vi "SW_Load_settings_to_main_tab_2.vi"(0 "Settings path in":path, 2 "Researcher name":string="Researcher", 3 "error in (no error)":errorcluster) -> (6 "Settings cluster out":T1={"Defaults"={"Default User"=0.0, "VISA Resource Name "=""}, "Recording and saving"={"Researcher name"="", "Name prefix"="", "Data filtering"=0, "Stop at"=0.0, "\"Stop at\" enabled"=FALSE}, "Geometry"={"Cage diameter, mm"=0, "Starting angle MIDFIELD"=0, "Starting angle BORDER"=0, "Radius, mm CENTER"=0, "Radius, mm MIDFIELD"=0, "N segments MIDFIELD"=0, "N segments BORDER"=0, "R-gap, mm"=0.0, "Bridge swap"=FALSE, "Bridge H. offset"=0.0, "Bridge V. offset"=0.0, "Twisted neck"=FALSE}, "IO parameters"={"IO general config."=0, "IO 1 configuration"=0, "IO 2 configuration"=0, "IO 3 configuration"=0, "IO 4 configuration"=0, "Activate ext. RS-232"=0, "IO inversion config."=0, "Sync capability"=1}, "Stimulus presets array"=[{"Event type"=0, "Dur., s"=0.0, "Stim., s"=0.0, "TTL out N"=1, "Set/Clear"=FALSE, "Stim. has been set"=FALSE}, {"Event type"=0, "Dur., s"=0.0, "Stim., s"=0.0, "TTL out N"=1, "Set/Clear"=FALSE, "Stim. has been set"=FALSE}, {"Event type"=0, "Dur., s"=0.0, "Stim., s"=0.0, "TTL out N"=1, "Set/Clear"=FALSE, "Stim. has been set"=FALSE}, {"Event type"=0, "Dur., s"=0.0, "Stim., s"=0.0, "TTL out N"=1, "Set/Clear"=FALSE, "Stim. has been set"=FALSE}, {"Event type"=0, "Dur., s"=0.0, "Stim., s"=0.0, "TTL out N"=1, "Set/Clear"=FALSE, "Stim. has been set"=FALSE}, {"Event type"=0, "Dur., s"=0.0, "Stim., s"=0.0, "TTL out N"=1, "Set/Clear"=FALSE, "Stim. has been set"=FALSE}, {"Event type"=0, "Dur., s"=0.0, "Stim., s"=0.0, "TTL out N"=1, "Set/Clear"=FALSE, "Stim. has been set"=FALSE}, {"Event type"=0, "Dur., s"=0.0, "Stim., s"=0.0, "TTL out N"=1, "Set/Clear"=FALSE, "Stim. has been set"=FALSE}, {"Event type"=0, "Dur., s"=0.0, "Stim., s"=0.0, "TTL out N"=1, "Set/Clear"=FALSE, "Stim. has been set"=FALSE}, {"Event type"=0, "Dur., s"=0.0, "Stim., s"=0.0, "TTL out N"=1, "Set/Clear"=FALSE, "Stim. has been set"=FALSE}, {"Event type"=0, "Dur., s"=0.0, "Stim., s"=0.0, "TTL out N"=1, "Set/Clear"=FALSE, "Stim. has been set"=FALSE}, {"Event type"=0, "Dur., s"=0.0, "Stim., s"=0.0, "TTL out N"=1, "Set/Clear"=FALSE, "Stim. has been set"=FALSE}, {"Event type"=0, "Dur., s"=0.0, "Stim., s"=0.0, "TTL out N"=1, "Set/Clear"=FALSE, "Stim. has been set"=FALSE}, {"Event type"=0, "Dur., s"=0.0, "Stim., s"=0.0, "TTL out N"=1, "Set/Clear"=FALSE, "Stim. has been set"=FALSE}], "Settings loaded OK"=FALSE} {"Stimulus presets array"."Event type" items=["Stay for N seconds"]; "Stimulus presets array"."TTL out N" items=["1"=1, "2"=2, "1+2"=3]; "Geometry"."Cage diameter, mm" scale=0.0..340.0}, 7 "Settings file path":path, 10 "error out":errorcluster={"status"=TRUE, "code"=1, "source"="Dequeue Element in NI_LVConfig.lvlib:Read Value Without Comment.vi->NI_LVConfig.lvlib:Read Key (I32).vi->SW_Load_settings_to_main_tab.vi"})   [LabVIEW 2018]
uses:
  Controls/CTL_Settings_cluster.ctl
  Controls/CTL_IO_params_cluster.ctl
  Controls/CTL_Single_stimulus_setting.ctl
  <vilib>/Utility/config.llb/NI_LVConfig.lvlib
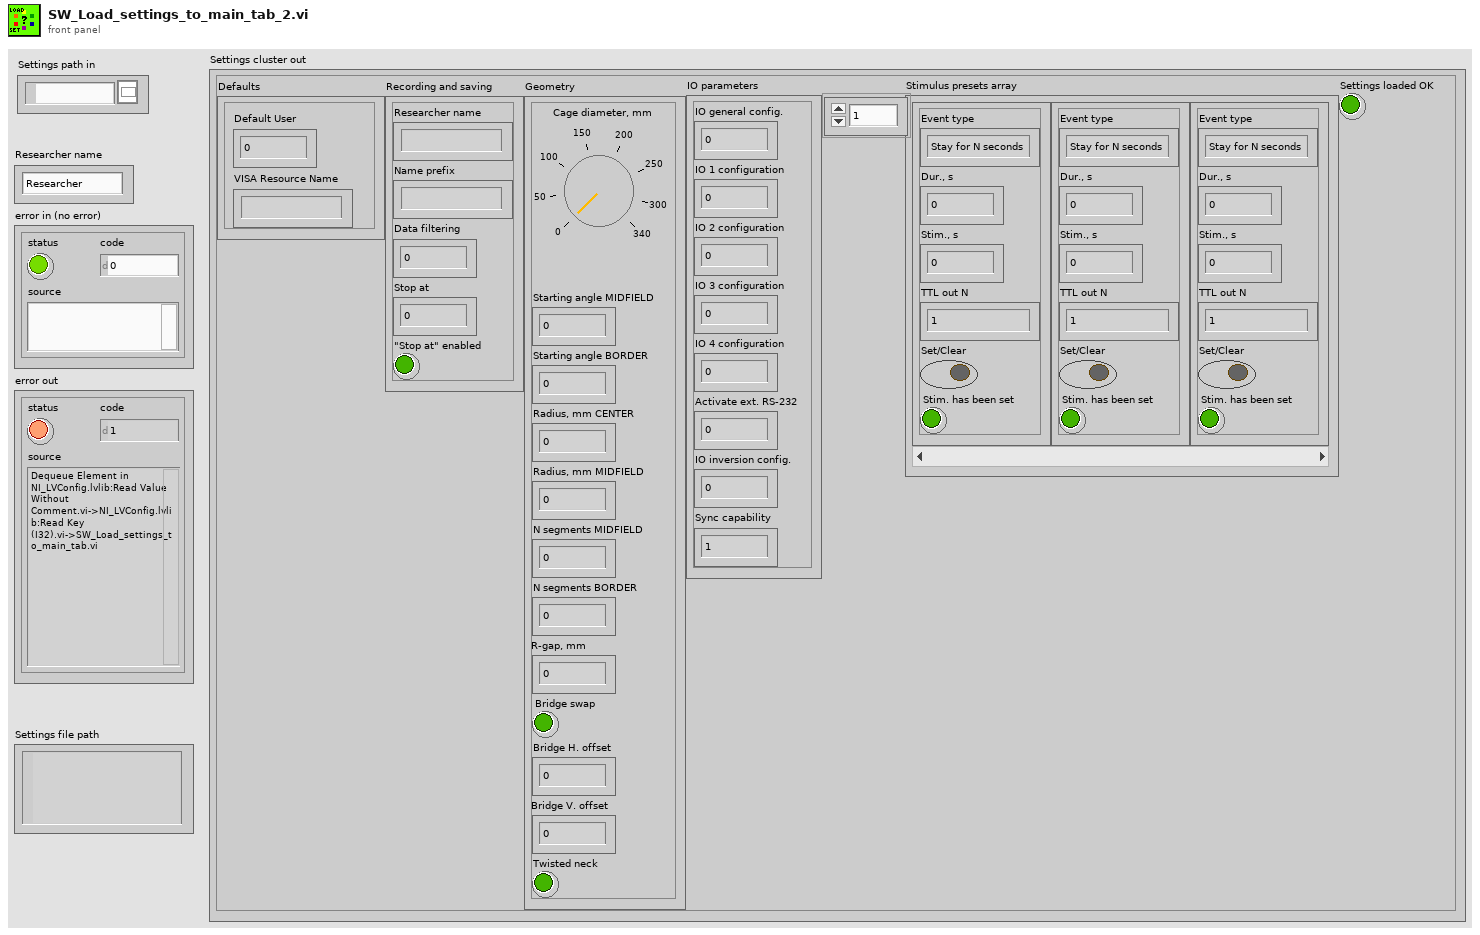
[diagram p1: front panel]
types:
  T1 = typedef "CTL_Settings_cluster.ctl" = cluster{"Defaults":cluster{"Default User":dbl, "VISA Resource Name ":string}, "Recording and saving":cluster{"Researcher name":string, "Name prefix":string, "Data filtering":u16, "Stop at":dbl, "\"Stop at\" enabled":bool}, "Geometry":cluster{"Cage diameter, mm":u16, "Starting angle MIDFIELD":i16, "Starting angle BORDER":i16, "Radius, mm CENTER":u16, "Radius, mm MIDFIELD":u16, "N segments MIDFIELD":u8, "N segments BORDER":u8, "R-gap, mm":sgl, "Bridge swap":bool, "Bridge H. offset":sgl, "Bridge V. offset":sgl, "Twisted neck":bool}, "IO parameters":T2, "Stimulus presets array":T3[], "Settings loaded OK":bool}
  T2 = typedef "CTL_IO_params_cluster.ctl" = cluster{"IO general config.":u16, "IO 1 configuration":u16, "IO 2 configuration":u16, "IO 3 configuration":u16, "IO 4 configuration":u16, "Activate ext. RS-232":u16, "IO inversion config.":u16, "Sync capability":u8}
  T3 = typedef "CTL_Single_stimulus_setting.ctl" = cluster{"Event type":u16, "Dur., s":sgl, "Stim., s":sgl, "TTL out N":u16, "Set/Clear":bool, "Stim. has been set":bool}
  T4 = typedef "NI_LVConfig.lvlib/Config Data RefNum.ctl" = refnum<k1>
  T5 = cluster{"Default User":dbl, "VISA Resource Name ":string}
  T6 = cluster{"Researcher name":string, "Name prefix":string, "Data filtering":u16, "Stop at":dbl, "\"Stop at\" enabled":bool}
  T7 = cluster{"Cage diameter, mm":u16, "Starting angle MIDFIELD":i16, "Starting angle BORDER":i16, "Radius, mm CENTER":u16, "Radius, mm MIDFIELD":u16, "N segments MIDFIELD":u8, "N segments BORDER":u8, "R-gap, mm":sgl, "Bridge swap":bool, "Bridge H. offset":sgl, "Bridge V. offset":sgl, "Twisted neck":bool}
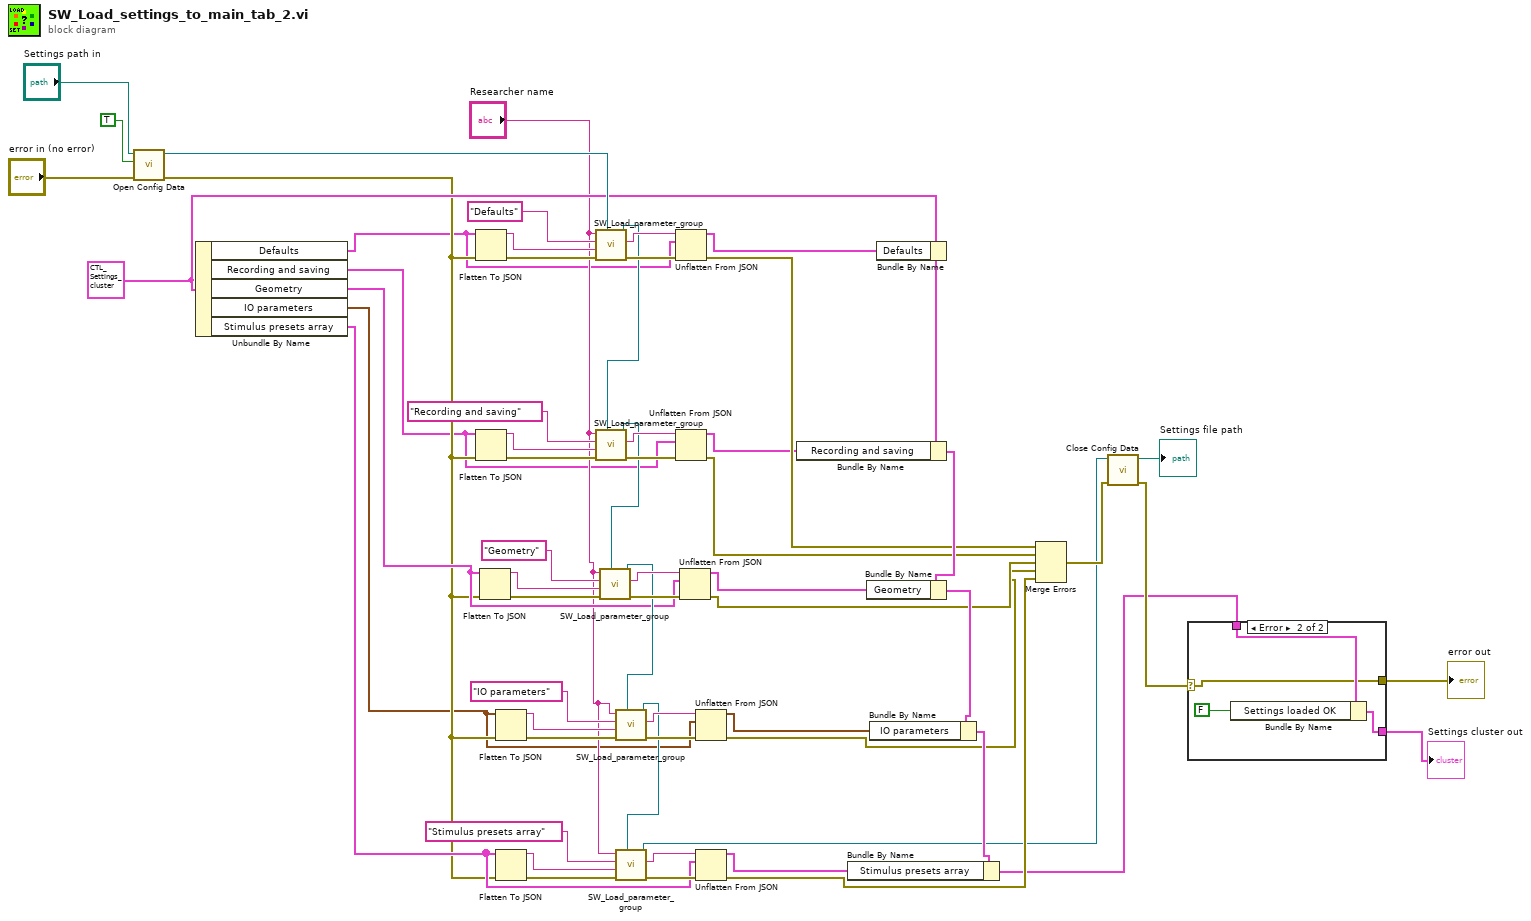
[diagram p0: block diagram]
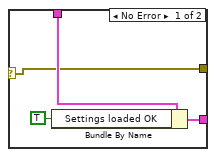
[diagram p2: hidden frame]
diagram:
  w39 = T1 {"Defaults"={"Default User"=0.0, "VISA Resource Name "="Tracker"}, "Recording and saving"={"Researcher name"="Researcher", "Name prefix"="Track", "Data filtering"=5, "Stop at"=0.0, "\"Stop at\" enabled"=FALSE}, "Geometry"={"Cage diameter, mm"=180, "Starting angle MIDFIELD"=0, "Starting angle BORDER"=0, "Radius, mm CENTER"=30, "Radius, mm MIDFIELD"=75, "N segments MIDFIELD"=2, "N segments BORDER"=4, "R-gap, mm"=0.0, "Bridge swap"=FALSE, "Bridge H. offset"=0.0, "Bridge V. offset"=0.0, "Twisted neck"=FALSE}, "IO parameters"={"IO general config."=12, "IO 1 configuration"=1, "IO 2 configuration"=1, "IO 3 configuration"=0, "IO 4 configuration"=0, "Activate ext. RS-232"=0, "IO inversion config."=0, "Sync capability"=1}, "Stimulus presets array"=[{"Event type"=0, "Dur., s"=0.0, "Stim., s"=0.0, "TTL out N"=1, "Set/Clear"=FALSE, "Stim. has been set"=FALSE}, {"Event type"=0, "Dur., s"=0.0, "Stim., s"=0.0, "TTL out N"=1, "Set/Clear"=FALSE, "Stim. has been set"=FALSE}, {"Event type"=0, "Dur., s"=0.0, "Stim., s"=0.0, "TTL out N"=1, "Set/Clear"=FALSE, "Stim. has been set"=FALSE}, {"Event type"=0, "Dur., s"=0.0, "Stim., s"=0.0, "TTL out N"=1, "Set/Clear"=FALSE, "Stim. has been set"=FALSE}, {"Event type"=0, "Dur., s"=0.0, "Stim., s"=0.0, "TTL out N"=1, "Set/Clear"=FALSE, "Stim. has been set"=FALSE}, {"Event type"=0, "Dur., s"=0.0, "Stim., s"=0.0, "TTL out N"=1, "Set/Clear"=FALSE, "Stim. has been set"=FALSE}, {"Event type"=0, "Dur., s"=0.0, "Stim., s"=0.0, "TTL out N"=1, "Set/Clear"=FALSE, "Stim. has been set"=FALSE}, {"Event type"=0, "Dur., s"=0.0, "Stim., s"=0.0, "TTL out N"=1, "Set/Clear"=FALSE, "Stim. has been set"=FALSE}, {"Event type"=0, "Dur., s"=0.0, "Stim., s"=0.0, "TTL out N"=1, "Set/Clear"=FALSE, "Stim. has been set"=FALSE}, {"Event type"=0, "Dur., s"=0.0, "Stim., s"=0.0, "TTL out N"=1, "Set/Clear"=FALSE, "Stim. has been set"=FALSE}, {"Event type"=0, "Dur., s"=0.0, "Stim., s"=0.0, "TTL out N"=1, "Set/Clear"=FALSE, "Stim. has been set"=FALSE}, {"Event type"=0, "Dur., s"=0.0, "Stim., s"=0.0, "TTL out N"=1, "Set/Clear"=FALSE, "Stim. has been set"=FALSE}, {"Event type"=0, "Dur., s"=0.0, "Stim., s"=0.0, "TTL out N"=1, "Set/Clear"=FALSE, "Stim. has been set"=FALSE}, {"Event type"=0, "Dur., s"=0.0, "Stim., s"=0.0, "TTL out N"=1, "Set/Clear"=FALSE, "Stim. has been set"=FALSE}], "Settings loaded OK"=FALSE} ("Settings cluster")
  n1 = call <vilib>:"Open Config Data.vi"("error in (no error)"="error in (no error)", "create file if necessary (T)"=TRUE, "configuration file path"="Settings path in") -> ("error out"=w6:errorcluster, "refnum"=w58:T4)  [unwired: 6 in, 1 out]
  n2 = Unbundle By Name(w39) -> ("Defaults"=w3:T5, "Recording and saving"=w2:T6, "Geometry"=w29:T7, "IO parameters"=w1:T2, "Stimulus presets array"=w21:T3[])
  n3 = Flatten To JSON(anything=w3, error in (no error)=w6) -> (JSON string=w57:string, 11:w55:errorcluster)  [unwired: 1 in]
  n4 = Flatten To JSON(anything=w2, error in (no error)=w6) -> (JSON string=w49:string, 11:w51:errorcluster)  [unwired: 1 in]
  n5 = Flatten To JSON(anything=w29, error in (no error)=w6) -> (JSON string=w45:string, 11:w43:errorcluster)  [unwired: 1 in]
  n6 = Flatten To JSON(anything=w1, error in (no error)=w6) -> (JSON string=w32:string, 11:w34:errorcluster)  [unwired: 1 in]
  n7 = Flatten To JSON(anything=w21, error in (no error)=w6) -> (JSON string=w26:string, 11:w24:errorcluster)  [unwired: 1 in]
  n8 = call "SW_Load_parameter_group.vi"("Settings file refnum in"=w58, "error in"=w55, "Default value (JSON)"=w57, "Group"="Defaults", "Researcher name"="Researcher name") -> ("error out"=w59:errorcluster, "Read value (JSON)"=w54:string, "Settings file refnum out"=w47:T4)  [unwired: 4 in]
  n9 = call "SW_Load_parameter_group.vi"("Settings file refnum in"=w47, "error in"=w51, "Default value (JSON)"=w49, "Group"="Recording and saving", "Researcher name"="Researcher name") -> ("error out"=w48:errorcluster, "Read value (JSON)"=w52:string, "Settings file refnum out"=w40:T4)  [unwired: 4 in]
  n10 = call "SW_Load_parameter_group.vi"("Settings file refnum in"=w40, "error in"=w43, "Default value (JSON)"=w45, "Group"="Geometry", "Researcher name"="Researcher name") -> ("error out"=w46:errorcluster, "Read value (JSON)"=w42:string, "Settings file refnum out"=w30:T4)  [unwired: 4 in]
  n11 = call "SW_Load_parameter_group.vi"("Settings file refnum in"=w30, "error in"=w34, "Default value (JSON)"=w32, "Group"="IO parameters", "Researcher name"="Researcher name") -> ("error out"=w31:errorcluster, "Read value (JSON)"=w35:string, "Settings file refnum out"=w19:T4)  [unwired: 4 in]
  n12 = call "SW_Load_parameter_group.vi"("Settings file refnum in"=w19, "error in"=w24, "Default value (JSON)"=w26, "Group"="Stimulus presets array", "Researcher name"="Researcher name") -> ("error out"=w27:errorcluster, "Read value (JSON)"=w23:string, "Settings file refnum out"=w8:T4)  [unwired: 4 in]
  n13 = Unflatten From JSON(JSON string=w54, type and defaults=w3, error in (no error)=w59) -> (value=w53:T5, error out=w18:errorcluster)  [unwired: 4 in]
  n14 = Unflatten From JSON(JSON string=w52, type and defaults=w2, error in (no error)=w48) -> (value=w5:T6, error out=w17:errorcluster)  [unwired: 4 in]
  n15 = Unflatten From JSON(JSON string=w42, type and defaults=w29, error in (no error)=w46) -> (value=w41:T7, error out=w16:errorcluster)  [unwired: 4 in]
  n16 = Unflatten From JSON(JSON string=w35, type and defaults=w1, error in (no error)=w31) -> (value=w36:T2, error out=w15:errorcluster)  [unwired: 4 in]
  n17 = Unflatten From JSON(JSON string=w23, type and defaults=w21, error in (no error)=w27) -> (value=w22:T3[], error out=w14:errorcluster)  [unwired: 4 in]
  n18 = Bundle By Name(cluster=w39, "Defaults"=w53) -> (w38:T1)
  n19 = Bundle By Name(cluster=w38, "Recording and saving"=w5) -> (w37:T1)
  n20 = Bundle By Name(cluster=w37, "Geometry"=w41) -> (w28:T1)
  n21 = Bundle By Name(cluster=w28, "IO parameters"=w36) -> (w20:T1)
  n22 = Bundle By Name(cluster=w20, "Stimulus presets array"=w22) -> (w10:T1)
  n23 = Merge Errors(w18, w17, w16, w15, w14) -> (w13:errorcluster)
  n24 = call <vilib>:"Close Config Data.vi"("error in (no error)"=w13, "refnum"=w8) -> ("error out"=w12:errorcluster, "file path"=→"Settings file path":path)  [unwired: 8 in]
  n25 = case shown="Error" w12 {
    selector: w12 -> [w64 w68]
    tunnel: [w64 w68] -> w11
    tunnel: w10 -> [w66 w70]
    tunnel: [w63 w67] -> w9
    frame No Error {
      n26 = Bundle By Name(cluster=w66, "Settings loaded OK"=TRUE) -> (w63:T1)
    }
    frame Error {
      n27 = Bundle By Name(cluster=w70, "Settings loaded OK"=FALSE) -> (w67:T1)
    }
  }
  "Settings cluster out" <- w9
  "error out" <- w11
